vi "Global.vi"() -> ()   [LabVIEW 2020]
panel:
  in  "提示信息 2":refnum<vi>
  in  "电机安装":bool[](array[boolean])
  in  "控制器安装支架":bool[](array[boolean])
  in  "控制器支架":bool[](array[boolean])
  in  "硬件版本号":string
  in  "ECU前序显示字":refnum<vi>
  in  "电机前序显示字":refnum<vi>
  in  "MOTOR码":string
  in  "MOTOR追溯码":string
  in  "ECU码":string
  in  "ECU追溯码":string
  in  "ECU结果显示":refnum<vi>
  in  "ECU自动":refnum<vi>
  in  "确定":bool
  in  "产品型号":string(combo)="R128"
  in  "电机结果显示":refnum<vi>
  in  "result":string
  in  "检测结果":refnum<vi>
  in  "电机生产数量":refnum<vi>
  in  "安装支架生产数量":refnum<vi>
  out "模式":u32
  in  "更换产品":refnum<vi>
  in  "提示信息":refnum<vi>
  in  "电机程序自动":refnum<vi>
  in  "报警图标":refnum<vi>
  in  "程序关闭":bool
  in  "Info":refnum<vi>
  in  "Result":refnum<vi>
  in  "批次":refnum<vi>
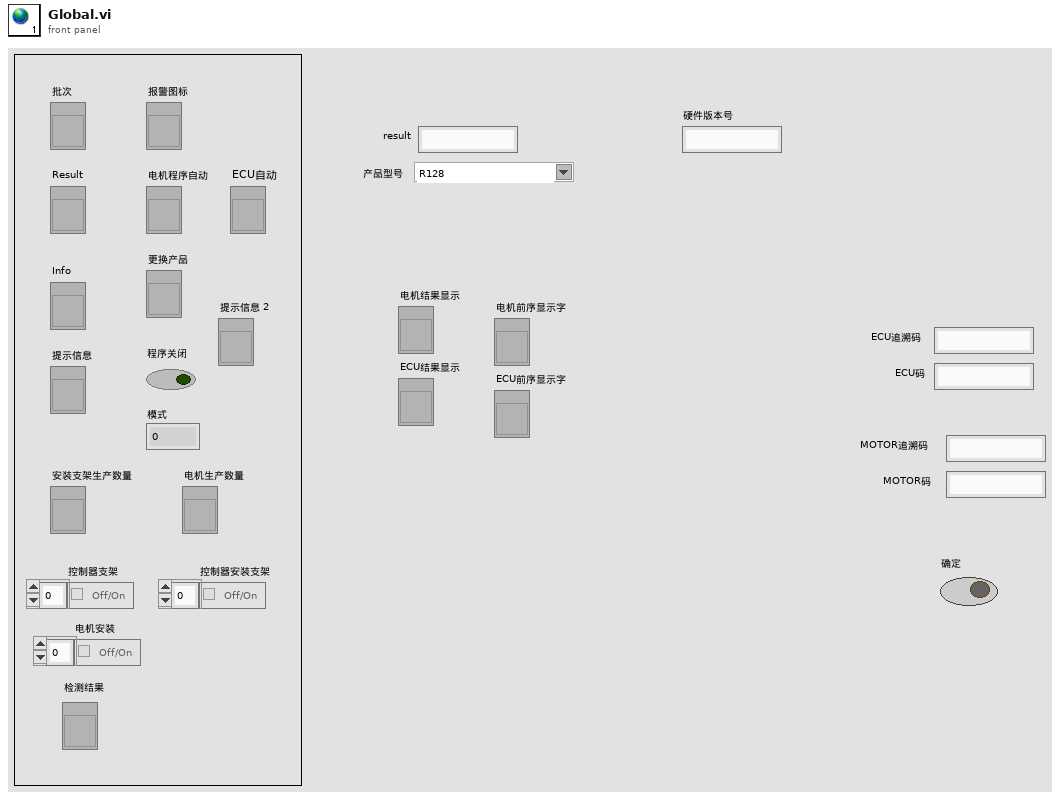
[diagram p1: front panel]
diagram:
